vi "External_Pause or Resume VIs.vi"(8 "error in":errorcluster, 9 "Action":enum16{"Pause", "Resume", "Toggle Pause"}(ring), 10 "VIs":string[](array[string])) -> (0 "error out":errorcluster, 1 "Symbol":i32[](array[numeric]), 2 "VIs":string[](array[string]))   [LabVIEW 2013]
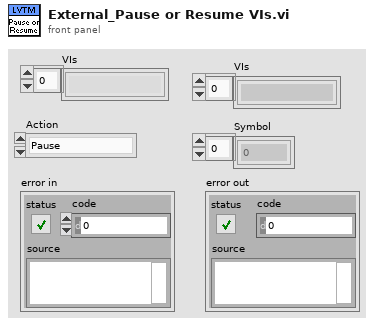
[diagram p1: front panel]
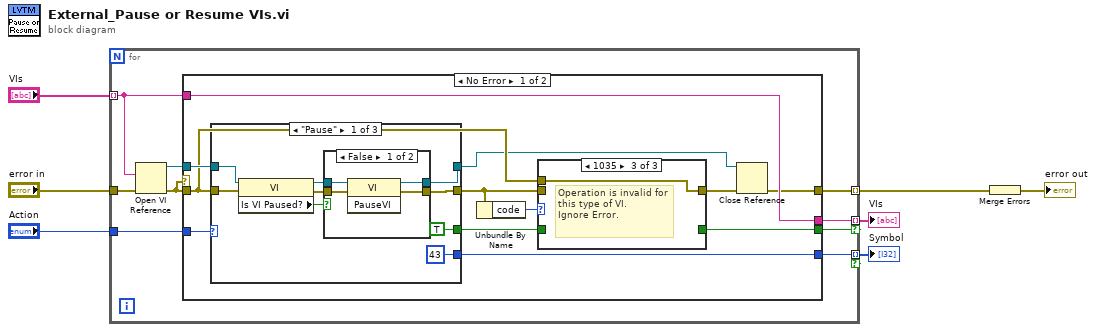
[diagram p0: block diagram]
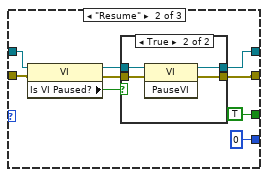
[diagram p5: hidden frame]
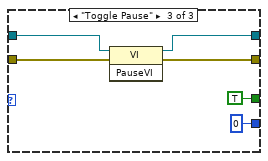
[diagram p7: hidden frame]
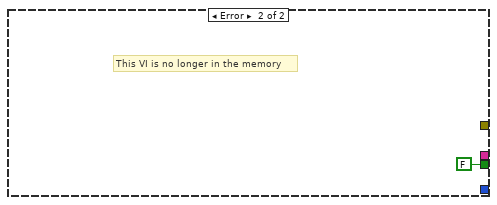
[diagram p8: hidden frame]
diagram:
  n1 = for {
    tunnel: "VIs" -> [w13] mode=indexing
    tunnel: "error in" -> [w15]
    tunnel: [w14] -> w3 mode=indexing
    tunnel: "Action" -> [w12]
    tunnel: [w10] -> w2 mode=indexing if=w8
    tunnel: [w9] -> w1 mode=indexing if=w8
    n2 = Open VI Reference(vi path=w13, error in (no error)=w15) -> (vi reference=w16:refnum<vi>, error out=w11:errorcluster)  [unwired: 4 out]
    n3 = case shown="No Error" w11 {
      tunnel: w16 -> [w28 _]
      tunnel: [w17 _] -> w14
      tunnel: w13 -> [w20 _]
      tunnel: w11 -> [w24 _]
      tunnel: w12 -> [w22 _]
      tunnel: [w20 _] -> w10
      tunnel: [w19 FALSE] -> w8
      tunnel: [w18 _] -> w9
      frame No Error {
        n4 = case shown="\"Pause\"" w22 {
          tunnel: w24 -> [w36 w51 w66]
          tunnel: w28 -> [w35 w50 w64]
          tunnel: [w33 w49 w63] -> w23
          tunnel: [w34 w48 w65] -> w25
          tunnel: [43 ("Active Item:Symbol Index") 0 ("Active Item:Symbol Index") 0 ("Active Item:Symbol Index")] -> w18
          tunnel: [TRUE TRUE TRUE] -> w21
          frame "Pause" {
            n5 = property class="VI"(reference=w35, error in=w36) -> (reference out=w37:refnum<vi>, error out=w38:errorcluster, "Is VI Paused?"=w39:bool)
            n6 = case shown="False" w39 {
              tunnel: [w45 w46] -> w34
              tunnel: [w44 w47] -> w33
              tunnel: w37 -> [w43 w47]
              tunnel: w38 -> [w42 w46]
              frame False {
                n7 = invoke class="VI" method="PauseVI"(reference=w43, error in=w42) -> (reference out=w44:refnum<vi>, error out=w45:errorcluster)  [unwired: 1 in, 1 out]
              }
              frame True {
              }
            }
          }
          frame "Resume" {
            n8 = property class="VI"(reference=w50, error in=w51) -> (reference out=w52:refnum<vi>, error out=w53:errorcluster, "Is VI Paused?"=w54:bool)
            n9 = case shown="True" w54 {
              tunnel: [w57 w62] -> w48
              tunnel: [w58 w61] -> w49
              tunnel: w52 -> [w58 w60]
              tunnel: w53 -> [w57 w59]
              frame False {
              }
              frame True {
                n10 = invoke class="VI" method="PauseVI"(reference=w60, error in=w59) -> (reference out=w61:refnum<vi>, error out=w62:errorcluster)  [unwired: 1 in, 1 out]
              }
            }
          }
          frame "Toggle Pause" {
            n11 = invoke class="VI" method="PauseVI"(reference=w64, error in=w66) -> (reference out=w63:refnum<vi>, error out=w65:errorcluster)  [unwired: 1 in, 1 out]
          }
        }
        n12 = Unbundle By Name(w25) -> ("code"=w27:i32)
        n13 = case shown="1035" w27 {
          tunnel: [w30 w31 w32] -> w26
          tunnel: w25 -> [w30 w31 _]
          tunnel: w24 -> [_ _ w32]
          tunnel: [w29 _ _] -> w19
          tunnel: w21 -> [w29 _ _]
          frame 0 {
          }
          frame Default {
          }
          frame 1035 {
            # "Operation is invalid for this type of VI.\nIgnore Error."
          }
        }
        n14 = Close Reference(reference=w23, error in (no error)=w26) -> (error out=w17:errorcluster)
      }
      frame Error {
        # "This VI is no longer in the memory"
      }
    }
  }
  "VIs" <- w2
  "Symbol" <- w1
  n15 = Merge Errors(w3) -> (→"error out":errorcluster)
